vi "Read Elevator Command.vi"(6 "Reset Idle State":bool, 8 "Button Cluster":T2, 9 "Axes":dbl[](array[numeric]), 10 "Driver Buttons":bool[](array[boolean])) -> (0 "Idle Mode":T1, 3 "Command":T3)   [LabVIEW 2014]
uses:
  Elevator Command.ctl
  Common Code/Elevator Idle Mode.ctl
  Real-Life Controls/Button Cluster.ctl
  Common Code/Elevator State.ctl
  Robot Global Data.vi
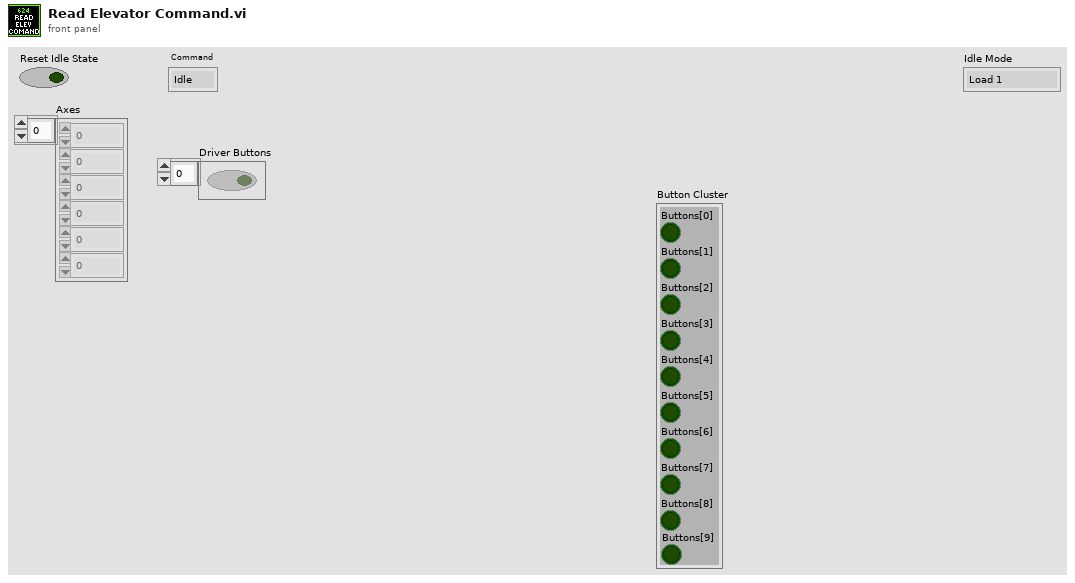
[diagram p1: front panel]
types:
  T1 = typedef "Elevator Idle Mode.ctl" = enum16{"Load 1", "Load 2", "Load 3", "Load Can", "Untip Can", "Step Load", "Drop Stack"}
  T2 = typedef "Button Cluster.ctl" = cluster{"Buttons[0]":bool, "Buttons[1]":bool, "Buttons[2]":bool, "Buttons[3]":bool, "Buttons[4]":bool, "Buttons[5]":bool, "Buttons[6]":bool, "Buttons[7]":bool, "Buttons[8]":bool, "Buttons[9]":bool}
  T3 = typedef "Elevator Command.ctl" = enum16{"Idle", "Load 1", "Load 2", "Load 3", "Drop Stack", "Eject Stack", "Untip Trashcan", "Load Trashcan", "HP Load"}
  T4 = typedef "Elevator State.ctl" = enum16{"Idle", "Goto Load Position", "Wait for Load", "Load Drop", "Load Lift", "Drop Stack", "Goto Eject Position", "Eject ", "Raise Trashcan", "Open Stabilizer", "Untip Drop", "Untip Wait", "Untip Lift", "Abort Load", "HP Load Wait", "HP Load Drop", "HP Load Lift", "HP Load Abort", "Close Stabilizer", "HP Load Lift First Tote", "HP Load Drop First Tote", "HP Load Finish"}
  T5 = typedef "Elevator Status.ctl" = cluster{"Height":dbl, "Enc Value":dbl, "Limit Override":bool, "Mode":T6, "High IR":bool, "Motor Out":dbl, "Ping Detect":bool, "Auto Elevator Indicators":T7, "Master Current":dbl, "Slave Current":dbl, "High Current":bool, "Current Tripped":bool, "Top Limit":bool, "Bottom Limit":bool, "Eject Piston":bool, "Stabilizer":bool, "Finger":bool, "Finger Height":dbl, "Finger Raw":dbl}
  T6 = typedef "Elevator Mode.ctl" = enum16{"Manual", "Safe", "Auto"}
  T7 = typedef "Auto Elevator Indicators.ctl" = cluster{"Target Out":dbl, "Storing Trashcan?":bool, "State":T4, "In Range":bool, "Store Can Command":bool, "HP Load":bool}
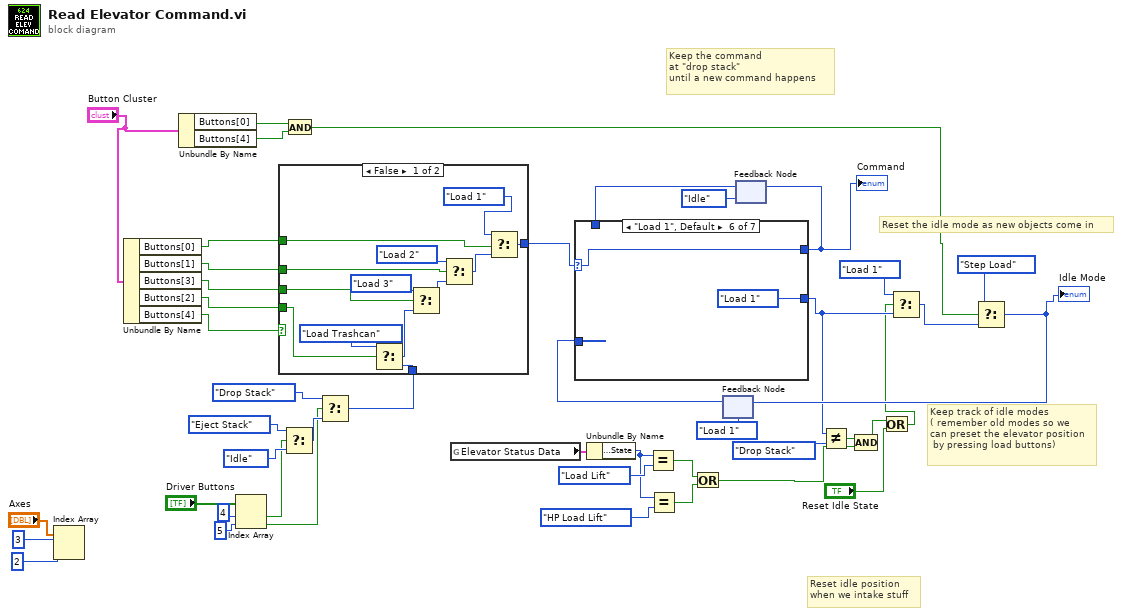
[diagram p0: block diagram]
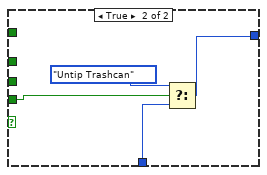
[diagram p2: hidden frame]
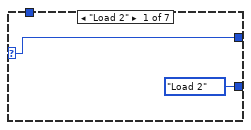
[diagram p3: hidden frame]
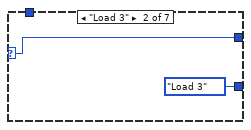
[diagram p4: hidden frame]
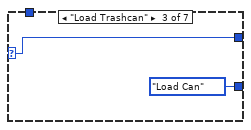
[diagram p5: hidden frame]
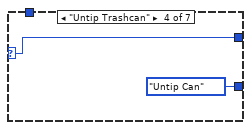
[diagram p6: hidden frame]
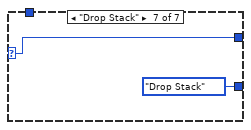
[diagram p9: hidden frame]
diagram:
  # "Reset idle position\nwhen we intake stuff"
  # "Keep track of idle modes\n( remember old modes so we\ncan preset the elevator position\n by pressing load buttons)"
  # "Keep the command\nat \"drop stack\"\nuntil a new command happens"
  # "Reset the idle mode as new objects come in"
  n1 = Index Array(array="Axes", index #1=3 ("index"), index #2=2 ("index")) -> ()  [unwired: 2 out]
  n2 = Unbundle By Name("Button Cluster") -> ("Buttons[0]"=w14:bool, "Buttons[1]"=w13:bool, "Buttons[3]"=w12:bool, "Buttons[2]"=w11:bool, "Buttons[4]"=w17:bool)
  n3 = Unbundle By Name("Button Cluster") -> ("Buttons[0]"=w31:bool, "Buttons[4]"=w30:bool)
  n4 = Index Array(array="Driver Buttons", index #1=4 ("index"), index #2=5 ("index")) -> (element #1=w19:bool, element #2=w15:bool)
  n5 = Select(t=Elevator_Command."Eject Stack", s=w19, f=Elevator_Command."Idle" ("t")) -> (s? t:f=w43:T3)
  n6 = And(x=w31, y=w30) -> (x .and. y?=w29:bool)
  n7 = Select(t=Elevator_Command."Drop Stack", s=w15, f=w43) -> (s? t:f=w16:T3)
  n8 = case shown="False" w17 {
    tunnel: w16 -> [w51 w61]
    tunnel: [w50 w60] -> w36
    tunnel: w14 -> [w49 _]
    tunnel: w13 -> [w48 _]
    tunnel: w12 -> [w47 _]
    tunnel: w11 -> [w46 w59]
    frame False {
      n9 = Select(t=Elevator_Command."Load Trashcan", s=w46, f=w51) -> (s? t:f=w57:T3)
      n10 = Select(t=Elevator_Command."Load 3", s=w47, f=w57) -> (s? t:f=w53:T3)
      n11 = Select(t=Elevator_Command."Load 2", s=w48, f=w53) -> (s? t:f=w52:T3)
      n12 = Select(t=Elevator_Command."Load 1", s=w49, f=w52) -> (s? t:f=w50:T3)
    }
    frame True {
      n13 = Select(t=Elevator_Command."Untip Trashcan", s=w59, f=w61) -> (s? t:f=w60:T3)
    }
  }
  n14 = global read "Robot Global Data.vi" "Elevator Status Data"() -> (w10:T5)
  n15 = Unbundle By Name(w10) -> ("Auto Elevator Indicators.State"=w7:T4)
  n16 = Equal?(x=w7, y=Elevator_State."Load Lift") -> (x = y?=w6:bool)
  n17 = Equal?(x=w7, y=Elevator_State."HP Load Lift") -> (x = y?=w4:bool)
  n18 = Or(x=w6, y=w4) -> (x .or. y?=w5:bool)
  n19 = feedback #1(Elevator_Idle_Mode."Load 1" ("Idle Mode")) -> (w35:T1)
  n20 = feedback #2(Elevator_Command."Idle" ("t")) -> (w21:T3)
  n21 = case shown="\"Load 1\", Default" w36 {
    selector: w36 -> [w63 w65 w67 w69 w72 w77 w79]
    tunnel: [Elevator_Idle_Mode."Load 2" ("Idle Mode") Elevator_Idle_Mode."Load 3" ("Idle Mode") Elevator_Idle_Mode."Load Can" ("Idle Mode") Elevator_Idle_Mode."Untip Can" ("Idle Mode") w74 Elevator_Idle_Mode."Load 1" ("Idle Mode") Elevator_Idle_Mode."Drop Stack" ("Idle Mode")] -> w23
    tunnel: w35 -> [_ _ _ _ w74 _ _]
    tunnel: [w63 w65 w67 w69 w71 w77 w79] -> w22
    tunnel: w21 -> [_ _ _ _ w73 _ _]
    frame "Load 2" {
    }
    frame "Load 3" {
    }
    frame "Load Trashcan" {
    }
    frame "Untip Trashcan" {
    }
    frame "Idle" {
      n22 = case shown="\"Drop Stack\"" w73 {
        selector: w73 -> [_ w76]
        tunnel: w72 -> [w75 _]
        tunnel: [w75 w76] -> w71
        frame "Idle", Default {
        }
        frame "Drop Stack" {
        }
      }
    }
    frame "Load 1", Default {
    }
    frame "Drop Stack" {
    }
  }
  "Command" <- w22
  n23 = feedback-in #2(w22) -> ()
  n24 = Not Equal?(x=w23, y=Elevator_Idle_Mode."Drop Stack") -> (x != y?=w24:bool)
  n25 = Compound Arithmetic op=AND(w24, w5) -> (w2:bool)
  n26 = Or(x=w2, y="Reset Idle State") -> (x .or. y?=w1:bool)
  n27 = Select(t=Elevator_Idle_Mode."Load 1", s=w1, f=w23) -> (s? t:f=w28:T1)
  n28 = Select(t=Elevator_Idle_Mode."Step Load", s=w29, f=w28) -> (s? t:f=w26:T1)
  "Idle Mode" <- w26
  n29 = feedback-in #1(w26) -> ()
